vi "6.vi"() -> ()   [LabVIEW 2017]
panel:
  out "波形图":dbl[](graph)
  out "最小值":dbl
  out "最大值":dbl
  out "平均数":dbl
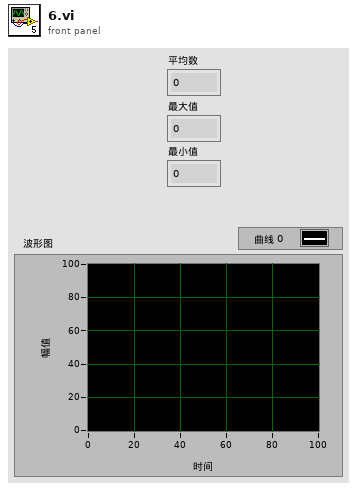
[diagram p1: front panel]
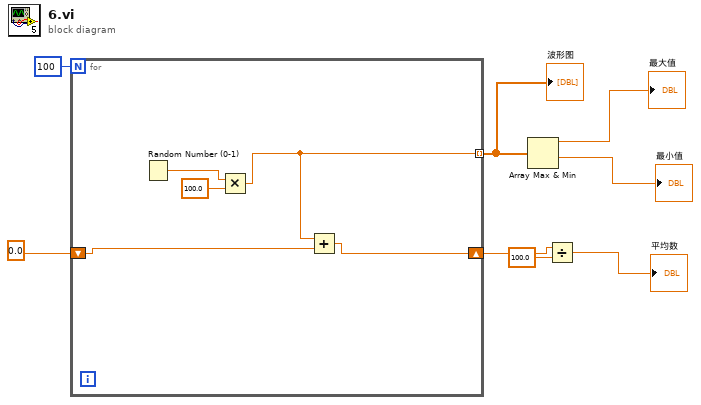
[diagram p0: block diagram]
diagram:
  n1 = for {
    N: 100 -> [_]
    tunnel: [w11] -> w1 mode=indexing
    shift-right: [w9] -> w6
    shift-left: 0.0 -> [w10]
    n2 = Random Number (0-1)() -> (number: 0 to 1=w12:dbl)
    n3 = Multiply(x=w12, y=100.0) -> (x*y=w11:dbl)
    n4 = Add(x=w11, y=w10) -> (x+y=w9:dbl)
  }
  "波形图" <- w1
  n5 = Array Max & Min(array=w1) -> (max value=→"最大值":dbl, min value=→"最小值":dbl)  [unwired: 2 out]
  n6 = Divide(x=w6, y=100.0) -> (x/y=→"平均数":dbl)
